vi "test core.vi"   [LabVIEW 2014]
uses:
  <vilib>/rvi/XilinxIP/XIPIN_XNode/niFpgaXIPIN.xnode
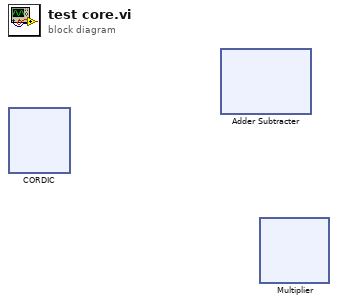
[diagram p0: block diagram]
diagram:
  n1 = xnode ("CORDIC")() -> ()
  n2 = xnode ("Adder Subtracter")() -> ()
  n3 = xnode ("Multiplier")() -> ()
